vi "AFG3352X.add services for 2nd channel.vi"(0 "i ref in":refnum<vi>, 3 "ms timeout (10000)":i32=10000, 5 "error in (no error)":errorcluster) -> (14 "i ref out":refnum<vi>, 17 "timed out":bool, 19 "error out":errorcluster)   [LabVIEW 2014, in "AFG3352X.lvlib"]
doc: "Declares the required DIM services."
uses:
  AFG3352X.lvlib
  CSlibraries-extern/DimLVEvent/LVDimInterface/LVDimInterface.lvlib
  CSCore/CSSystem/CSSystemLib/CSSystemLib.lvlib
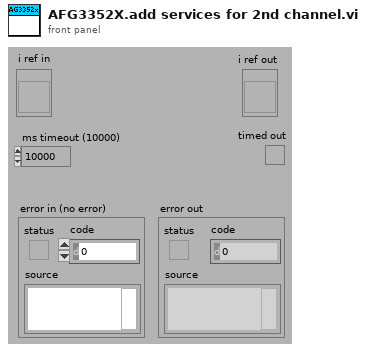
[diagram p1: front panel]
types:
  T1 = typedef "AFG3352X.lvlib/AFG3352X.i attribute.ctl" = cluster{"Act2ndValues":cluster{"frequency":dbl, "amplitude":dbl, "phase":dbl, "DCOffset":dbl, "waveformType":T2, "enableOutput":bool, "trigger":i16[], "serviceIDs":cluster{"frequencyID":i32, "amplitudeID":i32, "phaseID":i32, "DCOffsetID":i32, "waveformTypeID":i32, "enableOutputID":i32, "triggerID":i32}, "waveform":cluster{"data":waveform(dbl), "gain":dbl, "offset":dbl, "repetitionRate":dbl, "sampleRate":dbl}}, "Nom2ndValues":cluster{"frequency":dbl, "amplitude":dbl, "phase":dbl, "DCOffset":dbl, "waveformType":T2, "enableOutput":bool, "trigger":i16[], "serviceIDs":cluster{"frequencyID":i32, "amplitudeID":i32, "phaseID":i32, "DCOffsetID":i32, "waveformTypeID":i32, "enableOutputID":i32, "triggerID":i32}, "waveform":cluster{"data":waveform(dbl), "gain":dbl, "offset":dbl, "repetitionRate":dbl, "sampleRate":dbl}}, "DefaultChannel":i32, "ActAddValues":cluster{"Mode1":u16, "serviceIDs":cluster{"Mode1ID":i32, "Mode2ID":i32, "Burst1ID":i32, "Burst2ID":i32}, "Mode2":u16, "Burst1":i32, "Burst2":i32}, "NomAddValues":cluster{"Mode1":u16, "serviceIDs":cluster{"Mode1ID":i32, "Mode2ID":i32, "Burst1ID":i32, "Burst2ID":i32}, "Mode2 2":u16, "Burst1":i32, "Burst2":i32}, "enableBurstMode":bool}
  T2 = typedef "AFGBase.lvlib/AFGBase.waveformType.ctl" = enum16{"sine", "square", "ramp", "pulse", "noise", "DC", "arbitrary", "triangle", "ramp_up", "ramp_down", "amplitude modulation"}
  T3 = cluster{"my_serviceID":i32, "my_serviceID":i32, "my_serviceID":i32, "my_serviceID":i32, "my_serviceID":i32, "my_serviceID":i32, "my_serviceID":i32}
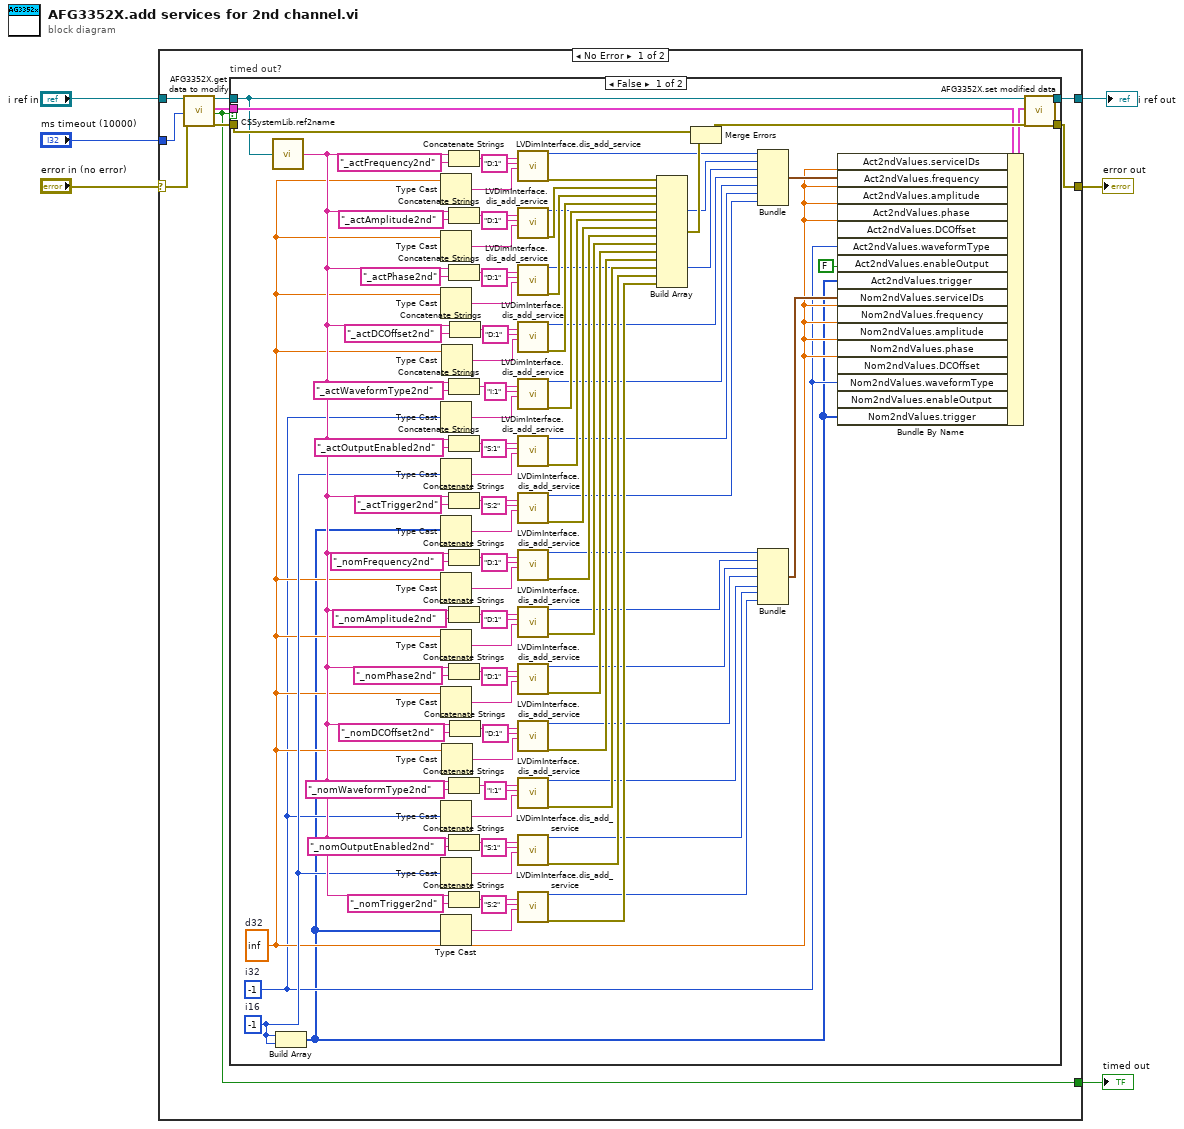
[diagram p0: block diagram]
diagram:
  n1 = case shown="No Error" "error in (no error)" {
    selector: "error in (no error)" -> [w13 w119]
    tunnel: [w9 w119] -> w5
    tunnel: "i ref in" -> [w15 w118]
    tunnel: [w11 w118] -> w1
    tunnel: "ms timeout (10000)" -> [w14 _]
    tunnel: [w8 _] -> w3
    frame No Error {
      n2 = call "AFG3352X.get data to modify.vi"("i ref in"=w15, "ms timeout (10000)"=w14, "error in (no error)"=w13) -> ("i ref out"=w12:refnum<vi>, "i attribute"=w7:T1, "timed out"=w8:bool, "error out"=w10:errorcluster)  [unwired: 13 in]
      n3 = case "timed out?" shown="False" w8 {
        tunnel: w12 -> [w23 w117]
        tunnel: [w115 w117] -> w11
        tunnel: w10 -> [w42 w116]
        tunnel: [w114 w116] -> w9
        tunnel: w7 -> [w39 _]
        frame False {
          w21 = i16 -1  # i16
          w19 = inf  # d32
          w17 = FALSE ("getValues.enableOutput")
          w18 = -1  # i32
          n4 = call "CSSystemLib.ref2name.vi"("obj refnum"=w23) -> ("name"=w57:string)
          n5 = Build Array(w21, w21) -> (w16:i16[])
          n6 = Type Cast(x=w19) -> (*(type *) &x=w110:string)  [unwired: 1 in]
          n7 = Type Cast(x=w19) -> (*(type *) &x=w109:string)  [unwired: 1 in]
          n8 = Type Cast(x=w19) -> (*(type *) &x=w102:string)  [unwired: 1 in]
          n9 = Type Cast(x=w18) -> (*(type *) &x=w94:string)  [unwired: 1 in]
          n10 = Type Cast(x=w21) -> (*(type *) &x=w90:string)  [unwired: 1 in]
          n11 = Type Cast(x=w16) -> (*(type *) &x=w86:string)  [unwired: 1 in]
          n12 = Type Cast(x=w19) -> (*(type *) &x=w82:string)  [unwired: 1 in]
          n13 = Type Cast(x=w19) -> (*(type *) &x=w81:string)  [unwired: 1 in]
          n14 = Type Cast(x=w19) -> (*(type *) &x=w74:string)  [unwired: 1 in]
          n15 = Type Cast(x=w18) -> (*(type *) &x=w66:string)  [unwired: 1 in]
          n16 = Type Cast(x=w21) -> (*(type *) &x=w62:string)  [unwired: 1 in]
          n17 = Type Cast(x=w16) -> (*(type *) &x=w58:string)  [unwired: 1 in]
          n18 = Type Cast(x=w19) -> (*(type *) &x=w98:string)  [unwired: 1 in]
          n19 = Type Cast(x=w19) -> (*(type *) &x=w70:string)  [unwired: 1 in]
          n20 = Concatenate Strings(w57, "_actFrequency2nd" ("string")) -> (w113:string)
          n21 = Concatenate Strings(w57, "_actAmplitude2nd" ("string")) -> (w106:string)
          n22 = Concatenate Strings(w57, "_actPhase2nd" ("string")) -> (w105:string)
          n23 = Concatenate Strings(w57, "_actWaveformType2nd" ("string")) -> (w97:string)
          n24 = Concatenate Strings(w57, "_actOutputEnabled2nd" ("string")) -> (w93:string)
          n25 = Concatenate Strings(w57, "_actTrigger2nd" ("string")) -> (w89:string)
          n26 = Concatenate Strings(w57, "_nomFrequency2nd" ("string")) -> (w85:string)
          n27 = Concatenate Strings(w57, "_nomAmplitude2nd" ("string")) -> (w78:string)
          n28 = Concatenate Strings(w57, "_nomPhase2nd" ("string")) -> (w77:string)
          n29 = Concatenate Strings(w57, "_nomWaveformType2nd" ("string")) -> (w69:string)
          n30 = Concatenate Strings(w57, "_nomOutputEnabled2nd" ("string")) -> (w65:string)
          n31 = Concatenate Strings(w57, "_nomTrigger2nd" ("string")) -> (w61:string)
          n32 = Concatenate Strings(w57, "_actDCOffset2nd" ("string")) -> (w101:string)
          n33 = Concatenate Strings(w57, "_nomDCOffset2nd" ("string")) -> (w73:string)
          n34 = call "LVDimInterface.dis_add_service.vi"("serviceName"=w113, "typeDescriptor"="D:1", "data"=w110) -> ("my_serviceID"=w38:i32, "error out"=w56:errorcluster)  [unwired: 15 in]
          n35 = call "LVDimInterface.dis_add_service.vi"("serviceName"=w106, "typeDescriptor"="D:1", "data"=w109) -> ("my_serviceID"=w37:i32, "error out"=w55:errorcluster)  [unwired: 15 in]
          n36 = call "LVDimInterface.dis_add_service.vi"("serviceName"=w105, "typeDescriptor"="D:1", "data"=w102) -> ("my_serviceID"=w36:i32, "error out"=w54:errorcluster)  [unwired: 15 in]
          n37 = call "LVDimInterface.dis_add_service.vi"("serviceName"=w101, "typeDescriptor"="D:1", "data"=w98) -> ("my_serviceID"=w35:i32, "error out"=w53:errorcluster)  [unwired: 15 in]
          n38 = call "LVDimInterface.dis_add_service.vi"("serviceName"=w97, "typeDescriptor"="I:1", "data"=w94) -> ("my_serviceID"=w34:i32, "error out"=w52:errorcluster)  [unwired: 15 in]
          n39 = call "LVDimInterface.dis_add_service.vi"("serviceName"=w93, "typeDescriptor"="S:1", "data"=w90) -> ("my_serviceID"=w33:i32, "error out"=w51:errorcluster)  [unwired: 15 in]
          n40 = call "LVDimInterface.dis_add_service.vi"("serviceName"=w89, "typeDescriptor"="S:2", "data"=w86) -> ("my_serviceID"=w32:i32, "error out"=w50:errorcluster)  [unwired: 15 in]
          n41 = call "LVDimInterface.dis_add_service.vi"("serviceName"=w85, "typeDescriptor"="D:1", "data"=w82) -> ("my_serviceID"=w31:i32, "error out"=w49:errorcluster)  [unwired: 15 in]
          n42 = call "LVDimInterface.dis_add_service.vi"("serviceName"=w78, "typeDescriptor"="D:1", "data"=w81) -> ("my_serviceID"=w30:i32, "error out"=w48:errorcluster)  [unwired: 15 in]
          n43 = call "LVDimInterface.dis_add_service.vi"("serviceName"=w77, "typeDescriptor"="D:1", "data"=w74) -> ("my_serviceID"=w29:i32, "error out"=w47:errorcluster)  [unwired: 15 in]
          n44 = call "LVDimInterface.dis_add_service.vi"("serviceName"=w73, "typeDescriptor"="D:1", "data"=w70) -> ("my_serviceID"=w28:i32, "error out"=w46:errorcluster)  [unwired: 15 in]
          n45 = call "LVDimInterface.dis_add_service.vi"("serviceName"=w69, "typeDescriptor"="I:1", "data"=w66) -> ("my_serviceID"=w27:i32, "error out"=w45:errorcluster)  [unwired: 15 in]
          n46 = call "LVDimInterface.dis_add_service.vi"("serviceName"=w65, "typeDescriptor"="S:1", "data"=w62) -> ("my_serviceID"=w26:i32, "error out"=w44:errorcluster)  [unwired: 15 in]
          n47 = call "LVDimInterface.dis_add_service.vi"("serviceName"=w61, "typeDescriptor"="S:2", "data"=w58) -> ("my_serviceID"=w25:i32, "error out"=w43:errorcluster)  [unwired: 15 in]
          n48 = Build Array(w56, w55, w54, w53, w52, w51, w50, w49, w48, w47, w46, w45, w44, w43) -> (w41:errorcluster[])
          n49 = Merge Errors(w42, w41) -> (w40:errorcluster)
          n50 = Bundle("my_serviceID"=w38, "my_serviceID"=w37, "my_serviceID"=w36, "my_serviceID"=w35, "my_serviceID"=w34, "my_serviceID"=w33, "my_serviceID"=w32) -> (w22:T3)  [unwired: 1 in]
          n51 = Bundle("my_serviceID"=w31, "my_serviceID"=w30, "my_serviceID"=w29, "my_serviceID"=w28, "my_serviceID"=w27, "my_serviceID"=w26, "my_serviceID"=w25) -> (w20:T3)  [unwired: 1 in]
          n52 = Bundle By Name(cluster=w39, "Act2ndValues.serviceIDs"=w22, "Act2ndValues.frequency"=w19, "Act2ndValues.amplitude"=w19, "Act2ndValues.phase"=w19, "Act2ndValues.DCOffset"=w19, "Act2ndValues.waveformType"=w18, "Act2ndValues.enableOutput"=w17, "Act2ndValues.trigger"=w16, "Nom2ndValues.serviceIDs"=w20, "Nom2ndValues.frequency"=w19, "Nom2ndValues.amplitude"=w19, "Nom2ndValues.phase"=w19, "Nom2ndValues.DCOffset"=w19, "Nom2ndValues.waveformType"=w18, "Nom2ndValues.enableOutput"=w17, "Nom2ndValues.trigger"=w16) -> (w24:T1)
          n53 = call "AFG3352X.set modified data.vi"("i ref in"=w23, "i attribute"=w24, "error in (no error)"=w40) -> ("i ref out"=w115:refnum<vi>, "error out"=w114:errorcluster)  [unwired: 15 in]
        }
        frame True {
        }
      }
    }
    frame Error {
    }
  }
  "error out" <- w5
  "timed out" <- w3
  "i ref out" <- w1
